vi "轮删字符串.vi"(1 "字符串":string) -> (0 "新字符串":string)   [LabVIEW 2015]
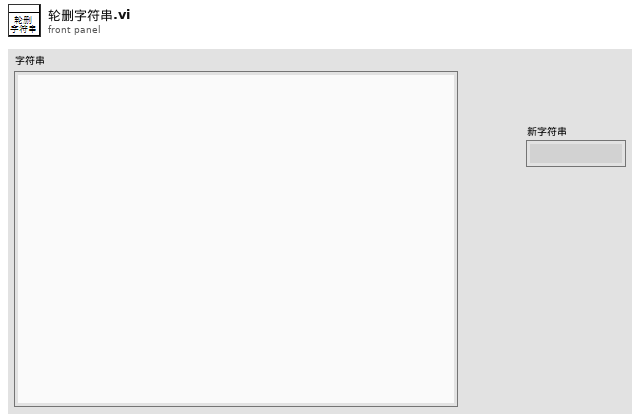
[diagram p1: front panel]
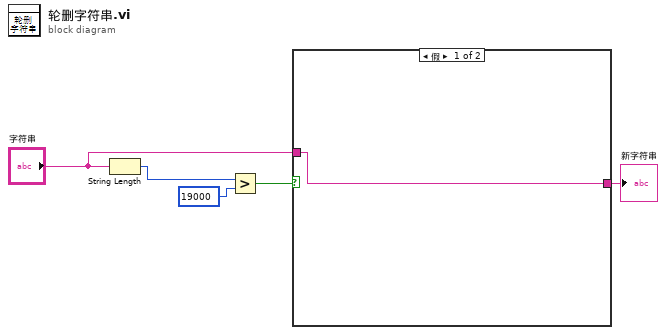
[diagram p0: block diagram]
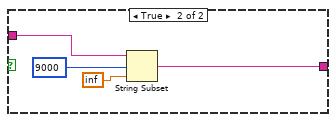
[diagram p2: hidden frame]
diagram:
  n1 = String Length(string="字符串") -> (length=w5:i32)
  n2 = Greater?(x=w5, y=19000) -> (0:w3:bool)
  n3 = case shown="假" w3 {
    tunnel: "字符串" -> [w6 w8]
    tunnel: [w6 w7] -> w1
    frame False {
    }
    frame True {
      n4 = String Subset(string=w8, offset (0)=9000, length (rest)=inf) -> (substring=w7:string)
    }
  }
  "新字符串" <- w1
